vi "Read move index.vi"(8 "error in (no error)":errorcluster, 11 "MotorSim in":refnum<class "MotorSim.lvclass">) -> (0 "error out":errorcluster, 2 "move index":i32, 3 "MotorSim out":refnum<class "MotorSim.lvclass">)   [LabVIEW 2018, in "MotorSim.lvclass"]
uses:
  MotorSim.lvclass
  MotorSim.lvclass/MotorSim.ctl
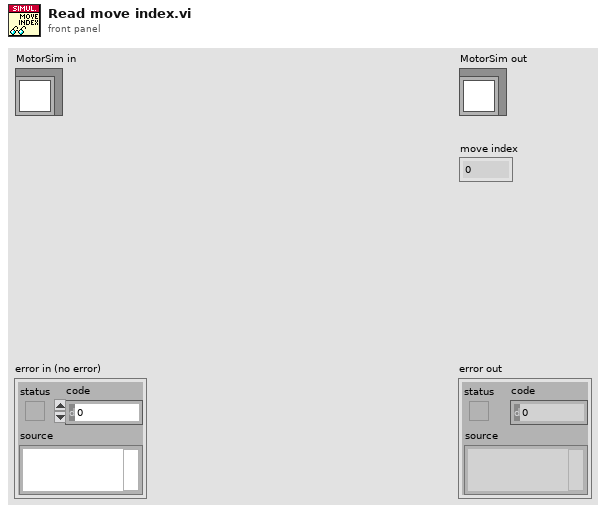
[diagram p1: front panel]
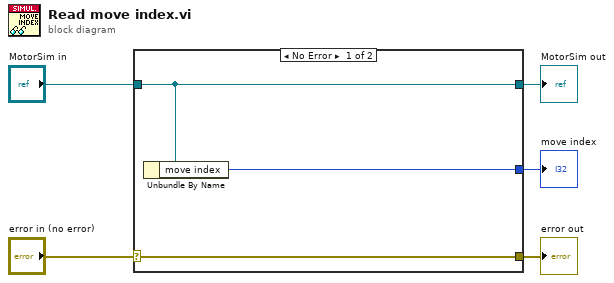
[diagram p0: block diagram]
diagram:
  n1 = case shown="No Error" "error in (no error)" {
    selector: "error in (no error)" -> [w8 w9]
    tunnel: [w8 w9] -> w4
    tunnel: [w7 w10] -> w2
    tunnel: "MotorSim in" -> [w7 w10]
    tunnel: [w6 _] -> w1
    frame No Error {
      n2 = Unbundle By Name(w7) -> ("move index"=w6:i32)
    }
    frame Error {
    }
  }
  "error out" <- w4
  "MotorSim out" <- w2
  "move index" <- w1
